vi "Double to Unix ns.vi"(3 "Timestamp":dbl) -> (1 "unix ns":i64)   [LabVIEW 2020, in "Vecto.lvlib"]
uses:
  Vecto.lvlib
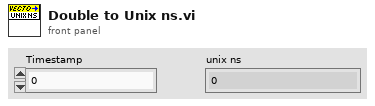
[diagram p1: front panel]
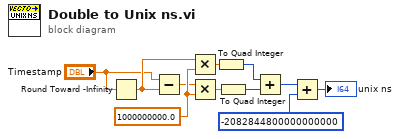
[diagram p0: block diagram]
diagram:
  w11 = 1000000000.0
  n1 = Round Toward -Infinity(1:"Timestamp") -> (0:w3:dbl)
  n2 = Subtract(x="Timestamp", y=w3) -> (x-y=w4:dbl)
  n3 = Multiply(x=w3, y=w11) -> (x*y=w5:dbl)
  n4 = Multiply(x=w4, y=w11) -> (x*y=w10:dbl)
  n5 = To Quad Integer(1:w5) -> (0:w2:i64)
  n6 = To Quad Integer(1:w10) -> (0:w9:i64)
  n7 = Add(x=w2, y=w9) -> (x+y=w8:i64)
  n8 = Add(x=w8, y=i64 -2082844800000000000) -> (x+y=→"unix ns":i64)
